vi "esp301 set backlash.vi"(7 "Seperator in":string, 8 "error in (no error)":errorcluster, 9 "Args":string[](array[string]), 10 "String":string, 11 "ESP301 in":refnum<class "ESP301.lvclass">) -> (0 "error out":errorcluster, 2 "new commands":string, 3 "ESP301 out":refnum<class "ESP301.lvclass">)   [LabVIEW 2020, in "ESP301.lvclass"]
uses:
  ESP301.lvclass
  ESP301.lvclass/ESP301.ctl
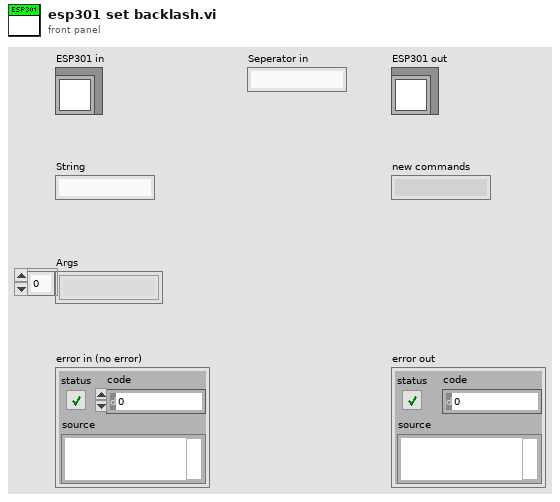
[diagram p1: front panel]
types:
  T1 = cluster{"Axis 1":cluster{"Value":dbl, "Min":dbl, "Max":dbl, "StepSize":dbl, "Tolerance":dbl, "ValueActual":dbl}, "Axis 2":cluster{"Value":dbl, "Min":dbl, "Max":dbl, "StepSize":dbl, "Tolerance":dbl, "ValueActual":dbl}, "Axis 3":cluster{"Value":dbl, "Min":dbl, "Max":dbl, "StepSize":dbl, "Tolerance":dbl, "ValueActual":dbl}}
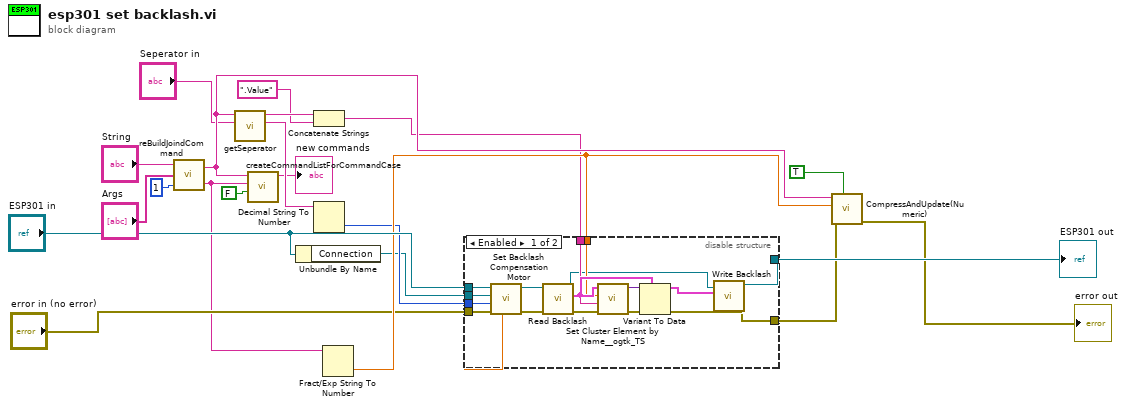
[diagram p0: block diagram]
diagram:
  n1 = call "reBuildJoindCommand.vi"("number of group elements (0)"=1, "Args"="Args", "Command 2"="String") -> ("Arg"=w14:string, "Command"=w15:string)
  n2 = call "getSeperator.vi"("Channel Seperator (\"\")"="Seperator in", "Command"=w15) -> ("Channel"=w10:string, "Seperator (e.g. \"Channel1\")"=w12:string)  [unwired: 8 in]
  n3 = call "createCommandListForCommandCase.vi"("immediate Check (only once)"=FALSE, "setvalue"=w14, "command"=w15) -> ("new commands"=→"new commands":string)  [unwired: 8 in]
  n4 = Unbundle By Name("ESP301 in") -> ("Connection"=w17:refnum<visa-resource-name>)
  n5 = Concatenate Strings(w12, ".Value" ("string")) -> (w13:string)
  n6 = Decimal String To Number(string=w10) -> (number=w18:i32)  [unwired: 2 in, 1 out]
  n7 = Fract/Exp String To Number(string=w14) -> (number=w19:dbl)  [unwired: 3 in, 1 out]
  n8 = disable-structure shown="Enabled" {
    disable-tunnel: [w37 w40] -> w21
    disable-tunnel: "ESP301 in" -> [w32 w40]
    disable-tunnel: w19 -> [w31 _]
    disable-tunnel: w18 -> [w30 _]
    disable-tunnel: w17 -> [w29 _]
    disable-tunnel: "error in (no error)" -> [w28 w39]
    disable-tunnel: w13 -> [w25 _]
    disable-tunnel: [w23 w39] -> w2
    frame Enabled {
      n9 = call-dynamic "Set Backlash Compensation Motor.vi"("Backlash Compensation Value (0 units)"=w31, "error in (no error)"=w28, "Axis (1)"=w30, "VISA resource name"=w29, "ESP301 in"=w32) -> ("error out"=w35:errorcluster, "ESP301 out"=w33:refnum<class "ESP301.lvclass">)  [unwired: 4 in, 1 out]
      n10 = call "Read Backlash.vi"("error in (no error)"=w35, "ESP301 in"=w33) -> ("error out"=w36:errorcluster, "Backlash"=w34:T1, "ESP301 out"=w22:refnum<class "ESP301.lvclass">)  [unwired: 7 in]
      n11 = call "Set Cluster Element by Name__ogtk_TS.vi"("error in (no error)"=w36, "Element Name (\"\": New Element Data Name)"=w25, "New Element Value"=w31, "Cluster"=w34) -> ("error out"=w26:errorcluster, "VCluster out"=w27:variant)  [unwired: 5 in, 1 out]
      n12 = Variant To Data(error in=w26, type=w34, Variant=w27) -> (data=w38:T1, error out=w24:errorcluster)
      n13 = call "Write Backlash.vi"("error in (no error)"=w24, "Backlash"=w38, "ESP301 in"=w22) -> ("error out"=w23:errorcluster, "ESP301 out"=w37:refnum<class "ESP301.lvclass">)  [unwired: 7 in]
    }
    frame Disabled {
    }
  }
  "ESP301 out" <- w21
  n14 = call "CompressAndUpdate(Numeric).vi"("force CVT update (false)"=TRUE ("force CVT update"), "error in"=w2, "Numeric"=w19, "command or variable name"=w15) -> ("error out"=→"error out":errorcluster)  [unwired: 7 in]
